vi "SweepLineTriggerWaveform.vi"(11 "digital waveform in":digitalwaveform(waveform)={"t0"=timestamp(0 s since 1904-01-01), "dt"=0.0, "Y"={"transitions"=[], "data"=[]}, "error"={"status"=FALSE, "code"=37421928, "source"=""}}) -> ()   [LabVIEW 2012]
uses:
  <vilib>/DAQmx/write.llb/DAQmx Write (Digital Wfm 1Chan NSamp).vi
  <vilib>/DAQmx/create/channels.llb/DAQmx Create Channel (CO-Pulse Generation-Frequency).vi
  <vilib>/DAQmx/create/channels.llb/DAQmx Create Channel (DO-Digital Output).vi
  <vilib>/Waveform/DWDTOps.llb/DWDT Digital Size.vi
  <vilib>/DAQmx/configure/timing.llb/DAQmx Timing (Sample Clock).vi
  <vilib>/DAQmx/configure/timing.llb/DAQmx Timing (Implicit).vi
  <vilib>/DAQmx/configure/trigger.llb/DAQmx Start Trigger (Digital Edge).vi
  <vilib>/Waveform/DWDTOps.llb/DWDT Uncompress Digital.vi
  <vilib>/DAQmx/miscellaneous.llb/DAQmx Fill In Error Info.vi
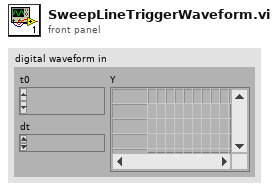
[diagram p1: front panel]
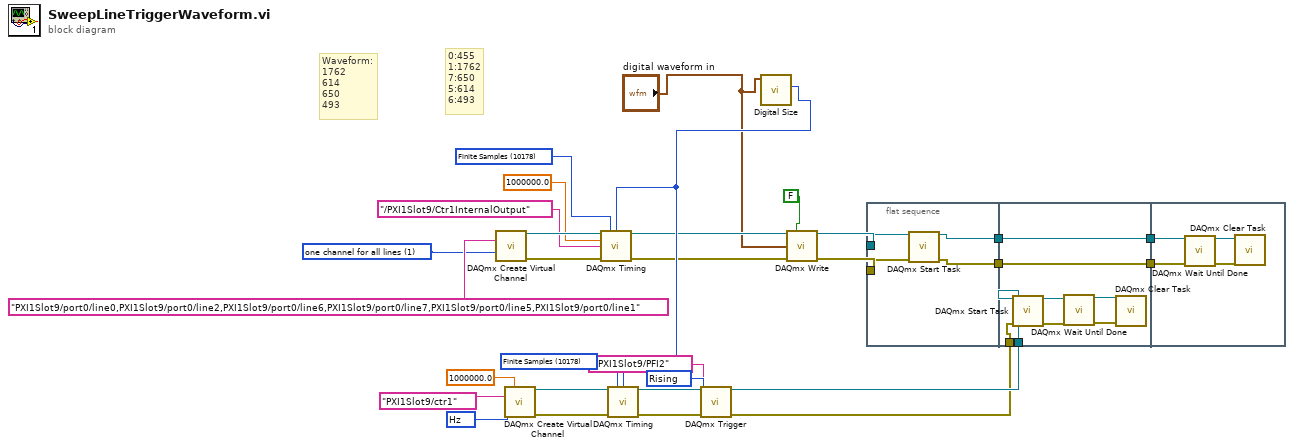
[diagram p0: block diagram]
diagram:
  w10 = 1 items=["one channel for each line", "one channel for all lines"] ("line grouping")
  w14 = 10178 items=["Finite Samples"=10178, "Continuous Samples"=10123, "Hardware Timed Single Point"=12522] ("sample mode")
  w21 = 10280 items=["Rising"=10280, "Falling"=10171] ("edge")
  w22 = 10178 items=["Finite Samples"=10178, "Continuous Samples"=10123, "Hardware Timed Single Point"=12522] ("sample mode")
  w28 = 10373 items=["Hz"=10373] ("units")
  # "0:455\n1:1762\n7:650\n5:614\n6:493"
  # "Waveform:\n1762\n614\n650\n493"
  n1 = call-poly <vilib>:"DAQmx Create Virtual Channel.vi"("lines"=tag "PXI1Slot9/port0/line0,PXI1Slot9/port0/line2,PXI1Slot9/port0/line6,PXI1Slot9/port0/line7,PXI1Slot9/port0/line5,PXI1Slot9/port0/line1", "line grouping"=w10) -> ("task out"=w18:refnum<k21>, "error out"=w17:errorcluster)  [unwired: 12 in]
  n2 = call-poly <vilib>:"DAQmx Create Virtual Channel.vi"("frequency"=1000000.0, "counter"=tag "PXI1Slot9/ctr1", "units"=w28) -> ("task out"=w27:refnum<k21>, "error out"=w24:errorcluster)  [unwired: 11 in]
  n3 = call-poly <vilib>:"Digital Size.vi"("digital waveform in"="digital waveform in") -> ("number of samples"=w23:i32)  [unwired: 7 in, 3 out]
  n4 = call-poly <vilib>:"DAQmx Timing.vi"("task/channels in"=w18, "sample mode"=w14, "samples per channel"=w23, "rate"=1000000.0, "source"=tag "/PXI1Slot9/Ctr1InternalOutput", "error in"=w17) -> ("task out"=w9:refnum<k21>, "error out"=w8:errorcluster)  [unwired: 8 in]
  n5 = call-poly <vilib>:"DAQmx Timing.vi"("task/channels in"=w27, "sample mode"=w22, "samples per channel"=w23, "error in"=w24) -> ("task out"=w26:refnum<k21>, "error out"=w25:errorcluster)  [unwired: 10 in]
  n6 = call-poly <vilib>:"DAQmx Trigger.vi"("task/channels in"=w26, "source"=tag "/PXI1Slot9/PFI2", "edge"=w21, "error in"=w25) -> ("task out"=w7:refnum<k21>, "error out"=w6:errorcluster)  [unwired: 10 in]
  n7 = call-poly <vilib>:"DAQmx Write.vi"("task/channels in"=w9, "auto start"=FALSE, "data"="digital waveform in", "error in"=w8) -> ("task out"=w12:refnum<k21>, "error out"=w11:errorcluster)  [unwired: 9 in, 1 out]
  n8 = flat-sequence {
    tunnel: w12 -> [w34]
    tunnel: w11 -> [w33]
    tunnel: [w32] -> w4
    tunnel: [w31] -> w2
    tunnel: w7 -> [w42]
    tunnel: w6 -> [w41]
    tunnel: [w40] -> w5
    tunnel: w4 -> [w40]
    tunnel: [w39] -> w3
    tunnel: w2 -> [w39]
    tunnel: w5 -> [w44]
    tunnel: w3 -> [w43]
    frame #0 {
      n9 = call <vilib>:"DAQmx Start Task.vi"("task/channels in"=w34, "error in"=w33) -> ("task out"=w32:refnum<k21>, "error out"=w31:errorcluster)  [unwired: 12 in]
    }
    frame #1 {
      n10 = call <vilib>:"DAQmx Start Task.vi"("task/channels in"=w42, "error in"=w41) -> ("task out"=w38:refnum<k21>, "error out"=w37:errorcluster)  [unwired: 12 in]
      n11 = call <vilib>:"DAQmx Wait Until Done.vi"("task/channels in"=w38, "error in"=w37) -> ("task out"=w35:refnum<k21>, "error out"=w36:errorcluster)  [unwired: 12 in]
      n12 = call <vilib>:"DAQmx Clear Task.vi"("task in"=w35, "error in"=w36) -> ()  [unwired: 13 in, 1 out]
    }
    frame #2 {
      n13 = call <vilib>:"DAQmx Wait Until Done.vi"("task/channels in"=w44, "error in"=w43) -> ("task out"=w46:refnum<k21>, "error out"=w45:errorcluster)  [unwired: 12 in]
      n14 = call <vilib>:"DAQmx Clear Task.vi"("task in"=w46, "error in"=w45) -> ()  [unwired: 13 in, 1 out]
    }
  }
